vi "Populate Single VI Help.vi"(6 "Show FP":bool, 7 "Force?(F)":bool, 8 "error in (no error)":errorcluster, 10 "VI Description":string, 11 "Path":path) -> (0 "error out":errorcluster)   [LabVIEW 2017, in "csmdoc.lvlib"]
uses:
  csmdoc.lvlib
  _Shared/CSM Shared.lvlib
  _tool/_file/csm-file-support.lvlib
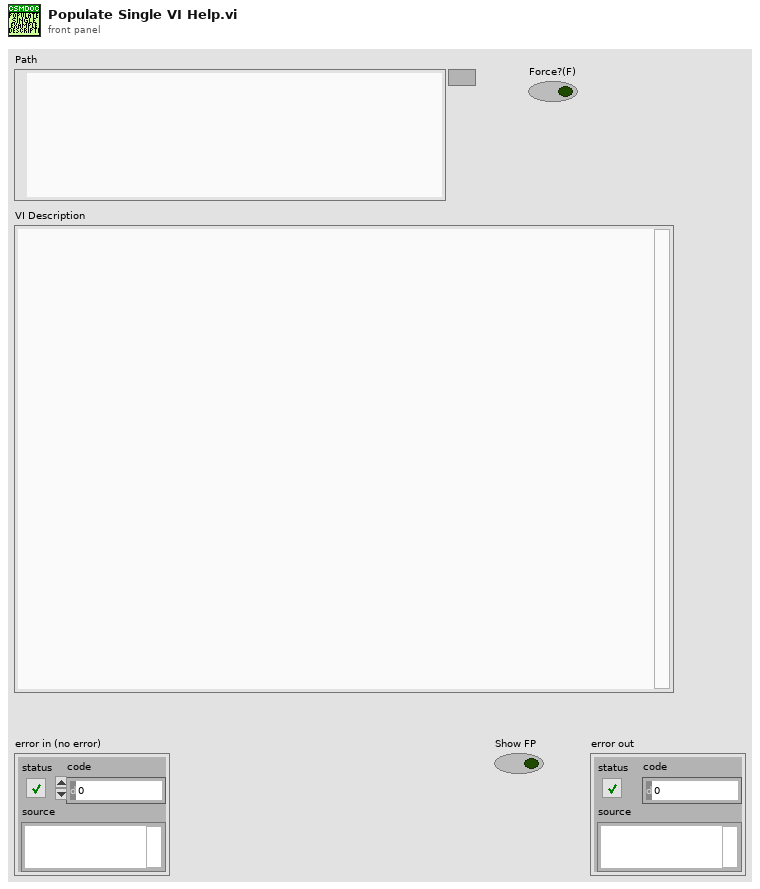
[diagram p1: front panel]
types:
  T1 = typedef "csmdoc.lvlib/DocElement.ctl" = cluster{"ID":string, "Content":string[], "SubIDs":string[], "Path":string[]}
  T2 = typedef "csmdoc.lvlib/DocNote.ctl" = cluster{"ID":string, "Content":string, "Type":string}
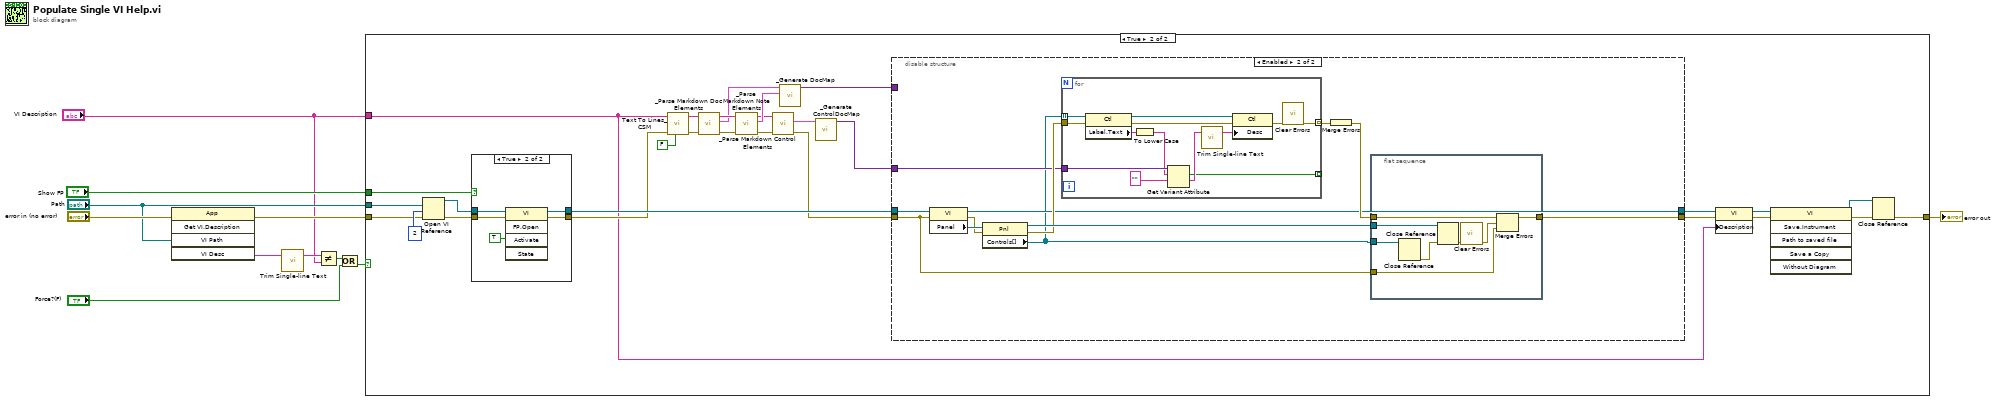
[diagram p0: block diagram]
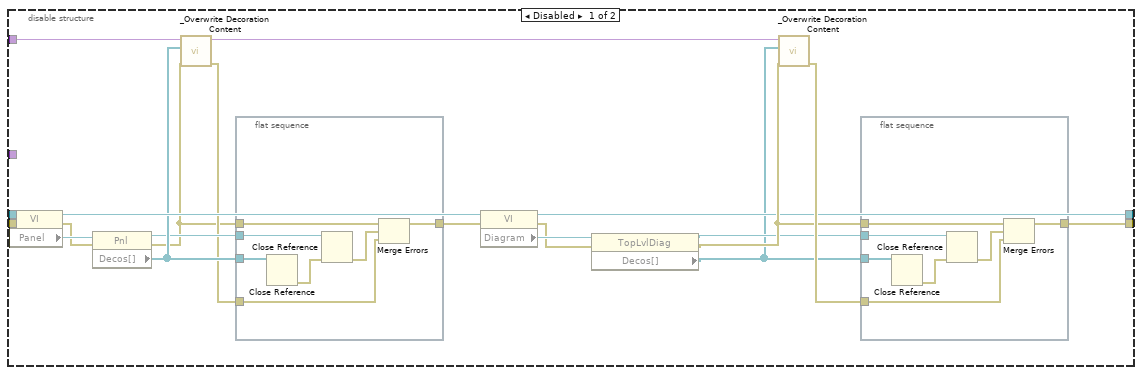
[diagram p3: hidden frame]
diagram:
  n1 = invoke class="App" method="Get VI.Description"(error in="error in (no error)", "VI Path"="Path") -> (error out=w11:errorcluster, "VI Desc"=w6:string)  [unwired: 3 in, 3 out]
  n2 = call "Trim Single-line Text.vi"("single-line text"=w6) -> ("trimed text"=w10:string)  [unwired: 2 in]
  n3 = Not Equal?(x=w10, y="VI Description") -> (x != y?=w2:bool)
  n4 = Or(x=w2, y="Force?(F)") -> (x .or. y?=w3:bool)
  n5 = case shown="True" w3 {
    tunnel: w11 -> [w12 w37]
    tunnel: "VI Description" -> [_ w22]
    tunnel: [w12 w34] -> w8
    tunnel: "Show FP" -> [_ w41]
    tunnel: "Path" -> [_ w33]
    frame False {
    }
    frame True {
      n6 = Open VI Reference(vi path=w33, options=2, error in (no error)=w37) -> (vi reference=w38:refnum<vi>, error out=w39:errorcluster)  [unwired: 3 in]
      n7 = case shown="True" w41 {
        tunnel: w39 -> [w109 w114]
        tunnel: w38 -> [w110 w113]
        tunnel: [w109 w112] -> w23
        tunnel: [w110 w111] -> w24
        frame False {
        }
        frame True {
          n8 = invoke class="VI" method="FP.Open"(reference=w113, error in=w114, "Activate"=TRUE ("Activate?")) -> (reference out=w111:refnum<vi>, error out=w112:errorcluster)  [unwired: 2 in, 3 out]
        }
      }
      n9 = call "Text To Lines_CSM.vi"("Remove Empty Lines? (T)"=FALSE ("Remove Empty Lines?(T)"), "error in (no error)"=w23, "String"=w22) -> ("error out"=w30:errorcluster, "Lines"=w31:string[])  [unwired: 7 in]
      n10 = call "_Parse Markdown Doc Elements.vi"("Error in"=w30, "Lines"=w31) -> ("Error out"=w28:errorcluster, "Array"=w27:T1[], "Lines (dup)"=w29:string[])  [unwired: 7 in]
      n11 = call "_Parse Markdown Note Elements.vi"("Error in"=w28, "Lines"=w29) -> ("Error out"=w16:errorcluster, "Array"=w26:T2[], "Lines (dup)"=w17:string[])  [unwired: 7 in]
      n12 = call "_Parse Markdown Control Elements.vi"("Error in"=w16, "Lines"=w17) -> ("Error out"=w15:errorcluster, "Array"=w14:T2[])  [unwired: 7 in, 1 out]
      n13 = call "_Generate DocMap.vi"("Array 2"=w26, "Array"=w27) -> ("Variant"=w25:variant)  [unwired: 9 in]
      n14 = call "_Generate ControlDocMap.vi"("Array"=w14) -> ("Variant"=w13:variant)  [unwired: 10 in]
      n15 = disable-structure shown="Enabled" {
        disable-tunnel: w15 -> [w59 w77]
        disable-tunnel: w25 -> [w54 _]
        disable-tunnel: w24 -> [w53 w86]
        disable-tunnel: [w44 w80] -> w21
        disable-tunnel: [w43 w81] -> w20
        disable-tunnel: w13 -> [_ w79]
        frame Disabled {
          n16 = property class="VI"(reference=w53, error in=w59) -> (reference out=w60:refnum<vi>, error out=w55:errorcluster, "Panel"=w61:refnum<vi>)
          n17 = property class="Pnl"(reference=w61, error in=w55) -> (reference out=w57:refnum<vi>, error out=w51:errorcluster, "Decos[]"=w58:refnum<vi>[])
          n18 = call "_Overwrite Decoration Content.vi"("error in (no error)"=w51, "Decos[]"=w58, "Variant in"=w54) -> ("error out"=w52:errorcluster, "Variant out"=w45:variant)  [unwired: 7 in]
          n19 = flat-sequence {
            tunnel: w58 -> [w75]
            tunnel: w57 -> [w74]
            tunnel: [w72] -> w56
            tunnel: w51 -> [w70]
            tunnel: w52 -> [w69]
            frame #0 {
              n20 = Close Reference(reference=w75) -> (error out=w73:errorcluster)  [unwired: 1 in]
              n21 = Close Reference(reference=w74, error in (no error)=w73) -> (error out=w71:errorcluster)
              n22 = Merge Errors(w70, w71, w69) -> (w72:errorcluster)
            }
          }
          n23 = property class="VI"(reference=w60, error in=w56) -> (reference out=w44:refnum<vi>, error out=w49:errorcluster, "Diagram"=w50:refnum<vi>)
          n24 = property class="TopLvlDiag"(reference=w50, error in=w49) -> (reference out=w46:refnum<vi>, error out=w47:errorcluster, "Decos[]"=w42:refnum<vi>[])
          n25 = call "_Overwrite Decoration Content.vi"("error in (no error)"=w47, "Decos[]"=w42, "Variant in"=w45) -> ("error out"=w48:errorcluster)  [unwired: 7 in, 1 out]
          n26 = flat-sequence {
            tunnel: w42 -> [w68]
            tunnel: w46 -> [w67]
            tunnel: [w65] -> w43
            tunnel: w47 -> [w63]
            tunnel: w48 -> [w62]
            frame #0 {
              n27 = Close Reference(reference=w68) -> (error out=w66:errorcluster)  [unwired: 1 in]
              n28 = Close Reference(reference=w67, error in (no error)=w66) -> (error out=w64:errorcluster)
              n29 = Merge Errors(w63, w64, w62) -> (w65:errorcluster)
            }
          }
        }
        frame Enabled {
          n30 = property class="VI"(reference=w86, error in=w77) -> (reference out=w80:refnum<vi>, error out=w76:errorcluster, "Panel"=w87:refnum<vi>)
          n31 = property class="Pnl"(reference=w87, error in=w76) -> (reference out=w85:refnum<vi>, error out=w82:errorcluster, "Controls[]"=w78:refnum<vi>[])
          n32 = for {
            tunnel: w78 -> [w108] mode=indexing
            tunnel: w82 -> [w107]
            tunnel: [w96] -> w84 mode=indexing
            tunnel: [w100] -> _ mode=indexing
            tunnel: w79 -> [w98]
            n33 = property class="Ctl"(reference=w108, error in=w107) -> (reference out=w106:refnum<vi>, error out=w105:errorcluster, "Label.Text"=w103:string)
            n34 = To Lower Case(string=w103) -> (all lower case string=w97:string)
            n35 = Get Variant Attribute(Variant=w98, name=w97, default value (empty Variant)="" ("regular expression")) -> (found=w100:bool, value=w101:string)  [unwired: 1 in, 2 out]
            n36 = call "Trim Single-line Text.vi"("single-line text"=w101) -> ("trimed text"=w99:string)  [unwired: 2 in]
            n37 = property class="Ctl"(reference=w106, error in=w105, "Desc"=w99) -> (error out=w104:errorcluster)  [unwired: 1 out]
            n38 = call <vilib>:"Clear Errors.vi"("error in (no error)"=w104) -> ("error out"=w96:errorcluster)  [unwired: 5 in, 1 out]
          }
          n39 = Merge Errors(w84) -> (w83:errorcluster)
          n40 = flat-sequence {
            tunnel: w78 -> [w95]
            tunnel: w85 -> [w94]
            tunnel: [w92] -> w81
            tunnel: w83 -> [w90]
            tunnel: w77 -> [w89]
            frame #0 {
              n41 = Close Reference(reference=w95) -> (error out=w93:errorcluster)  [unwired: 1 in]
              n42 = Close Reference(reference=w94, error in (no error)=w93) -> (error out=w91:errorcluster)
              n43 = call <vilib>:"Clear Errors.vi"("error in (no error)"=w91) -> ("error out"=w88:errorcluster)  [unwired: 5 in, 1 out]
              n44 = Merge Errors(w90, w88, w89) -> (w92:errorcluster)
            }
          }
        }
      }
      n45 = property class="VI"(reference=w21, error in=w20, "Description"=w22) -> (reference out=w18:refnum<vi>, error out=w19:errorcluster)
      n46 = invoke class="VI" method="Save.Instrument"(reference=w18, error in=w19) -> (reference out=w35:refnum<vi>, error out=w36:errorcluster)  [unwired: 4 in, 4 out]
      n47 = Close Reference(reference=w35, error in (no error)=w36) -> (error out=w34:errorcluster)
    }
  }
  "error out" <- w8
